vi "Test.vi"   [LabVIEW 2019]
doc: "This VI is called when test mode begins, and will automatically be terminated when it ends. You can add manual or automatic tests and invoke them from the dashboard."
uses:
  Robot Global Data.vi
  Diff_Drive_System/Diff_Drive_System_Globals.vi
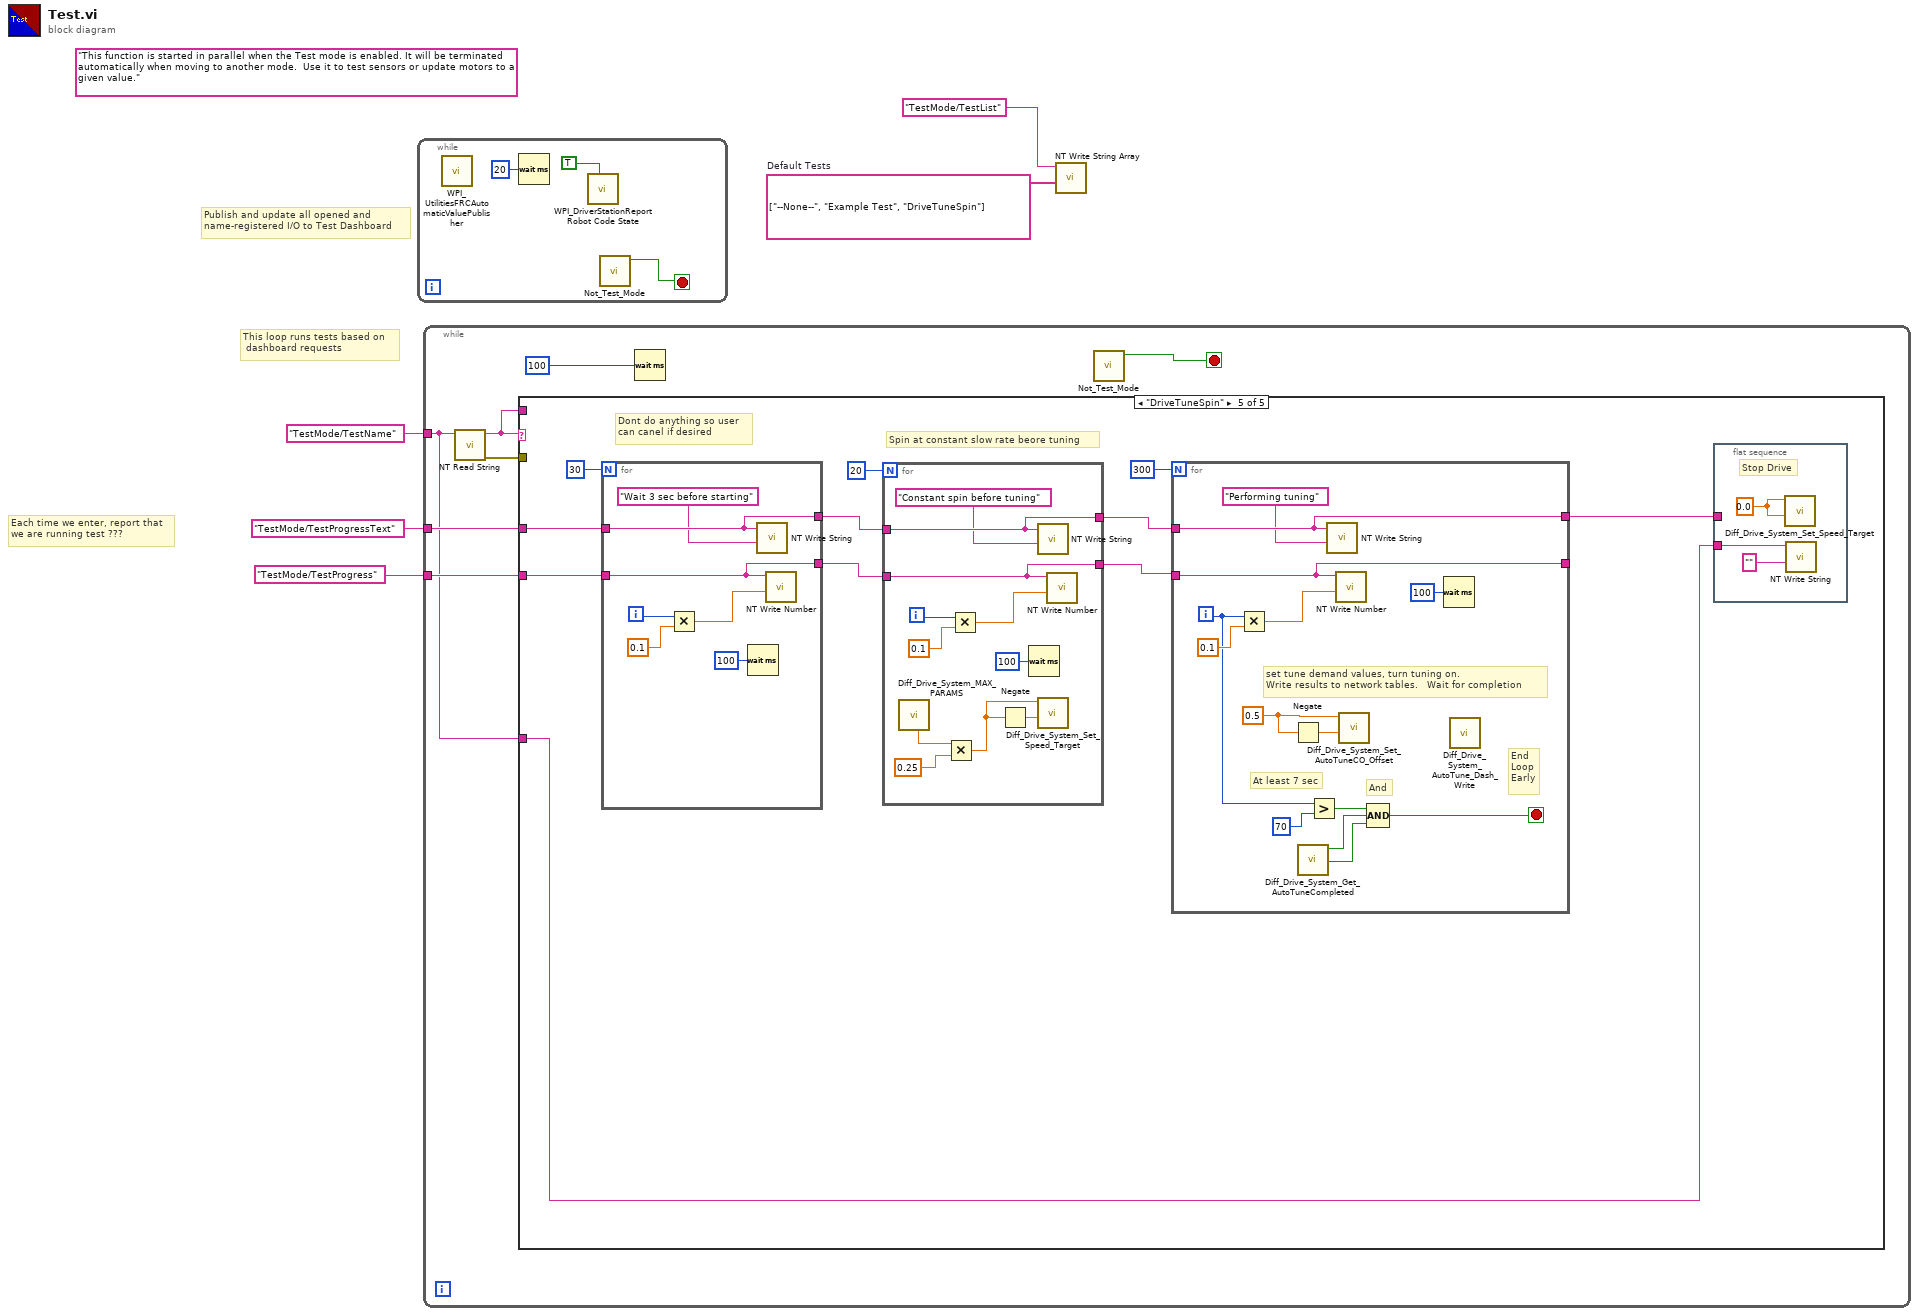
[diagram p0: block diagram]
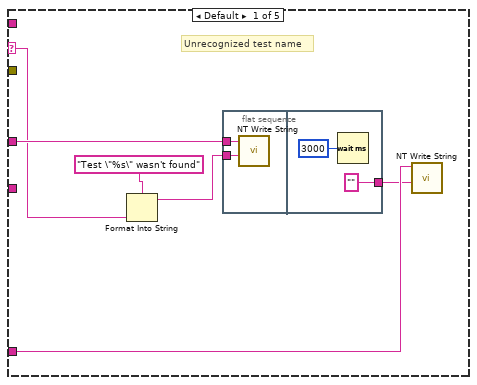
[diagram p2: hidden frame]
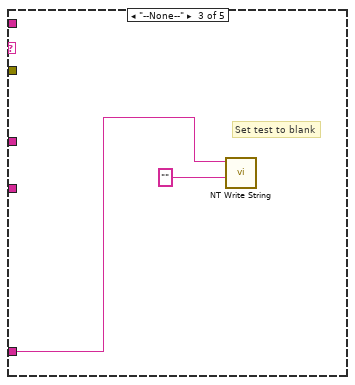
[diagram p4: hidden frame]
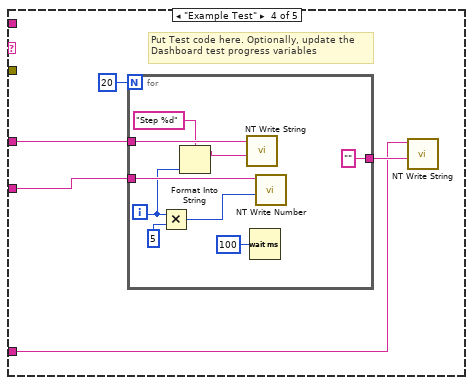
[diagram p5: hidden frame]
diagram:
  w2 = string[] ["--None--", "Example Test", "DriveTuneSpin"]  # Default Tests
  (unwired) "This function is started in parallel when the Test mode is enabled. It will be terminated automatically when moving to another mode.  Use it to test sensors or update motors to a given value."
  # "This loop runs tests based on \n dashboard requests"
  # "Publish and update all opened and\nname-registered I/O to Test Dashboard"
  # "Each time we enter, report that\nwe are running test ???"
  n1 = while {
    stop <- w6 stop-if-true
    n2 = call <vilib>:"WPI_UtilitiesFRCAutomaticValuePublisher.vi"() -> ()  [unwired: 12 in]
    n3 = Wait (ms)(milliseconds to wait=u32 20) -> ()  [unwired: 1 out]
    n4 = call <vilib>:"WPI_DriverStationReport Robot Code State.vi"("Test"=TRUE ("Autonomous")) -> ()  [unwired: 10 in, 1 out]
    n5 = call "Not_Test_Mode.vi"() -> ("NOT TEST MODE"=w6:bool)  [unwired: 11 in]
  }
  n6 = while {
    tunnel: "TestMode/TestName" ("Name") -> [w11]
    tunnel: "TestMode/TestProgressText" ("Name") -> [w14]
    tunnel: "TestMode/TestProgress" ("Name") -> [w13]
    stop <- w9 stop-if-true
    n7 = call <vilib>:"NT Read String.vi"("Name"=w11) -> ("error out"=w10:errorcluster, "String"=w12:string)  [unwired: 9 in]
    n8 = case shown="\"DriveTuneSpin\"" w12 {
      selector: w12 -> [w20 _ _ _ _]
      tunnel: w11 -> [w17 _ w27 w28 w42]
      tunnel: w14 -> [w21 _ _ w31 w51]
      tunnel: w13 -> [_ _ _ w32 w52]
      tunnel: w12 -> [_ _ _ _ _]
      tunnel: w10 -> [_ _ _ _ _]
      frame Default {
        # "Unrecognized test name"
        n9 = Format Into String(format string="Test \"%s\" wasn't found" ("Name"), w20) -> (resulting string=w19:string)  [unwired: 2 in, 1 out]
        n10 = flat-sequence {
          tunnel: w21 -> [w22]
          tunnel: w19 -> [w23]
          tunnel: ["" ("Name")] -> w16
          frame #0 {
            n11 = call <vilib>:"NT Write String.vi"("String"=w23, "Name"=w22) -> ()  [unwired: 9 in, 1 out]
          }
          frame #1 {
            n12 = Wait (ms)(milliseconds to wait=u32 3000) -> ()  [unwired: 1 out]
          }
        }
        n13 = call <vilib>:"NT Write String.vi"("String"=w16, "Name"=w17) -> ()  [unwired: 9 in, 1 out]
      }
      frame "" {
        # "No test to run"
      }
      frame "--None--" {
        # "Set test to blank"
        n14 = call <vilib>:"NT Write String.vi"("String"="" ("Name"), "Name"=w27) -> ()  [unwired: 9 in, 1 out]
      }
      frame "Example Test" {
        # "Put Test code here. Optionally, update the\nDashboard test progress variables"
        n15 = for {
          N: 20 -> [_]
          tunnel: w32 -> [w41]
          tunnel: w31 -> [w39]
          tunnel: ["" ("String")] -> w29
          i -> [w36]
          n16 = Multiply(x=w36, y=u32 5 ("milliseconds to wait")) -> (x*y=w37:u32)
          n17 = Format Into String(format string="Step %d", w36) -> (resulting string=w34:string)  [unwired: 2 in, 1 out]
          n18 = call <vilib>:"NT Write String.vi"("String"=w34, "Name"=w39) -> ()  [unwired: 9 in, 1 out]
          n19 = Wait (ms)(milliseconds to wait=u32 100) -> ()  [unwired: 1 out]
          n20 = call <vilib>:"NT Write Number.vi"("Numeric"=w37, "Name"=w41) -> ()  [unwired: 9 in, 1 out]
        }
        n21 = call <vilib>:"NT Write String.vi"("String"=w29, "Name"=w28) -> ()  [unwired: 9 in, 1 out]
      }
      frame "DriveTuneSpin" {
        # "Spin at constant slow rate beore tuning"
        # "Dont do anything so user\ncan canel if desired"
        n22 = for {
          N: 30 -> [_]
          tunnel: w52 -> [w82]
          tunnel: w51 -> [w83]
          tunnel: [w83] -> w48
          tunnel: [w82] -> w47
          i -> [w84]
          n23 = Multiply(x=w84, y=0.1) -> (x*y=w85:dbl)
          n24 = Wait (ms)(milliseconds to wait=u32 100) -> ()  [unwired: 1 out]
          n25 = call <vilib>:"NT Write String.vi"("String"="Wait 3 sec before starting" ("format string"), "Name"=w83) -> ()  [unwired: 9 in, 1 out]
          n26 = call <vilib>:"NT Write Number.vi"("Numeric"=w85, "Name"=w82) -> ()  [unwired: 9 in, 1 out]
        }
        n27 = for {
          N: 20 -> [_]
          tunnel: w47 -> [w75]
          tunnel: w48 -> [w76]
          tunnel: [w76] -> w45
          tunnel: [w75] -> w44
          i -> [w77]
          n28 = call "Diff_Drive_System_MAX_PARAMS.vi"() -> ("Max Drive Speed Ft/Sec"=w74:dbl)  [unwired: 9 in, 2 out]
          n29 = Multiply(x=w74, y=0.25) -> (x*y=w71:dbl)
          n30 = Multiply(x=w77, y=0.1) -> (x*y=w78:dbl)
          n31 = Negate(x=w71) -> (-x=w72:dbl)
          n32 = Wait (ms)(milliseconds to wait=u32 100) -> ()  [unwired: 1 out]
          n33 = call <vilib>:"NT Write String.vi"("String"="Constant spin before tuning" ("format string"), "Name"=w76) -> ()  [unwired: 9 in, 1 out]
          n34 = call "Diff_Drive_System_Set_Speed_Target.vi"("Right Speed Target FT/S"=w72, "Left Speed Target FT/S"=w71) -> ()  [unwired: 10 in]
          n35 = call <vilib>:"NT Write Number.vi"("Numeric"=w78, "Name"=w75) -> ()  [unwired: 9 in, 1 out]
        }
        n36 = for {
          N: 300 -> [_]
          tunnel: w44 -> [w65]
          tunnel: w45 -> [w66]
          tunnel: [w66] -> w43
          tunnel: [w65] -> _
          i -> [w61]
          stop <- w56 stop-if-true
          w63 = 0.5 ("Left CO Offset")
          # "End\nLoop\nEarly"
          # "And"
          # "At least 7 sec"
          # "set tune demand values, turn tuning on.\nWrite results to network tables.   Wait for completion"
          n37 = Multiply(x=w61, y=0.1) -> (x*y=w67:dbl)
          n38 = Negate(x=w63) -> (-x=w62:dbl)
          n39 = call "Diff_Drive_System_Get_AutoTuneCompleted.vi"() -> ("AutoTune Complete Right"=w57:bool, "AutoTune Complete Left"=w58:bool)  [unwired: 10 in]
          n40 = Greater?(x=w61, y=70) -> (0:w59:bool)
          n41 = call <vilib>:"NT Write String.vi"("String"="Performing tuning" ("format string"), "Name"=w66) -> ()  [unwired: 9 in, 1 out]
          n42 = call <vilib>:"NT Write Number.vi"("Numeric"=w67, "Name"=w65) -> ()  [unwired: 9 in, 1 out]
          n43 = call "Diff_Drive_System_Set_AutoTuneCO_Offset.vi"("Right CO Offset"=w62, "Left CO Offset"=w63) -> ()  [unwired: 10 in]
          n44 = Compound Arithmetic op=AND(w59, w58, w57) -> (w56:bool)
          n45 = Wait (ms)(milliseconds to wait=u32 100) -> ()  [unwired: 1 out]
          n46 = call "Diff_Drive_System_AutoTune_Dash_Write.vi"() -> ()  [unwired: 12 in]
        }
        n47 = flat-sequence {
          tunnel: w43 -> [_]
          tunnel: w42 -> [w54]
          frame #0 {
            w53 = 0.0 ("Left Speed Target FT/S")
            # "Stop Drive"
            n48 = call "Diff_Drive_System_Set_Speed_Target.vi"("Right Speed Target FT/S"=w53, "Left Speed Target FT/S"=w53) -> ()  [unwired: 10 in]
            n49 = call <vilib>:"NT Write String.vi"("String"="", "Name"=w54) -> ()  [unwired: 9 in, 1 out]
          }
        }
      }
    }
    n50 = Wait (ms)(milliseconds to wait=u32 100) -> ()  [unwired: 1 out]
    n51 = call "Not_Test_Mode.vi"() -> ("NOT TEST MODE"=w9:bool)  [unwired: 11 in]
  }
  n52 = call <vilib>:"NT Write String Array.vi"("String Array"=w2, "Name"="TestMode/TestList") -> ()  [unwired: 9 in, 1 out]
